vi "_Main_03.vi"() -> ()   [LabVIEW 2017]
uses:
  <vilib>/Instr/_visa.llb/VISA Configure Serial Port (Instr).vi
panel:
  out "Power LOG":cluster{dbl[], dbl[]}(graph)
  in  "Boolean":bool
  out "y":dbl
  in  "Set temp":dbl=195.0 min=195.0 max=395.0
  in  "OK Button":bool
  out "TrigTimer, s":dbl
  out "temp":dbl format="%#.2g"
  out "serv1":i32
  out "serv2":i32
  out "serv3":i32
  out "serv4":i32
  out "Vout, V":dbl format="%#.2g"
  out "Vin, V":dbl format="%#.3g"
  out "Temp, K":dbl
  out "Temp_sp, K":dbl
  out "Temp_gsp, K":dbl
  out "Temp LOG":cluster{dbl[], dbl[]}(graph)
  out "Bytes at Port":u32
  out "RecTry":i32
  in  "Stop Button":bool
  in  "COM port":refnum<visa-resource-name>
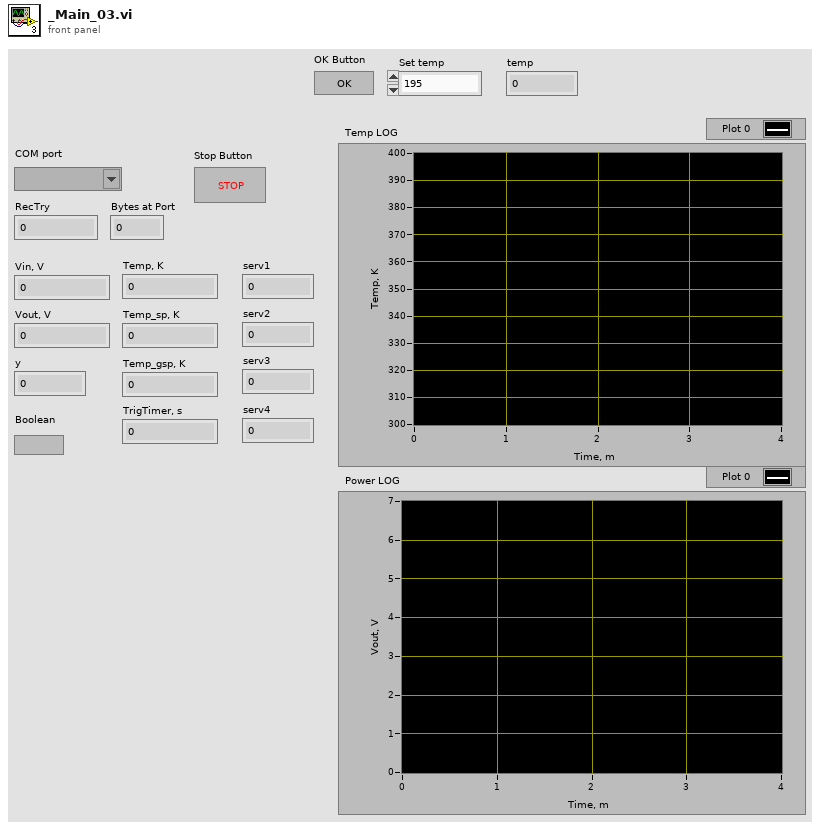
[diagram p1: front panel]
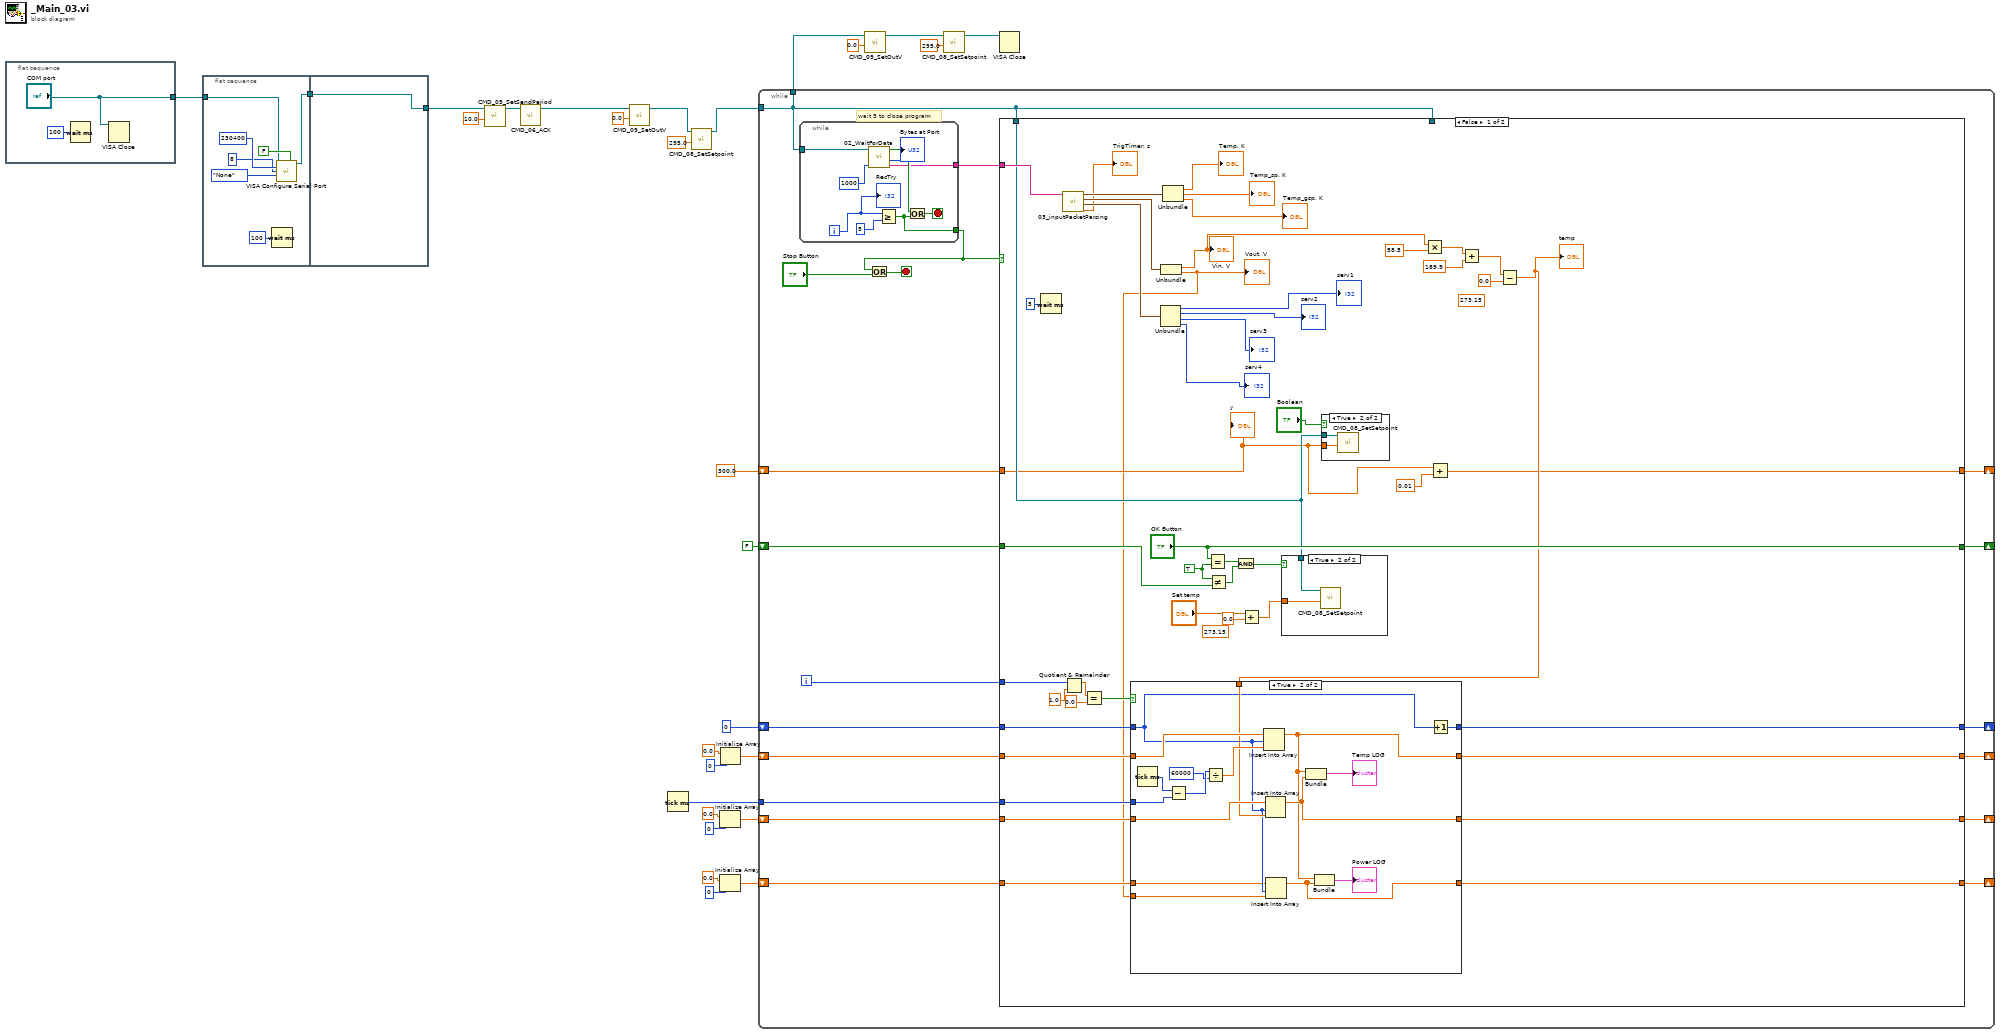
[diagram p0: block diagram]
diagram:
  n1 = flat-sequence {
    tunnel: ["COM port"] -> w28
    frame #0 {
      n2 = Wait (ms)(milliseconds to wait=u32 100) -> ()  [unwired: 1 out]
      n3 = VISA Close(VISA resource name="COM port") -> ()  [unwired: 1 in, 1 out]
    }
  }
  n4 = flat-sequence {
    tunnel: w28 -> [w33]
    tunnel: [w32] -> w25
    tunnel: [w38] -> w16
    tunnel: w25 -> [w38]
    frame #0 {
      n5 = Wait (ms)(milliseconds to wait=u32 100) -> ()  [unwired: 1 out]
      n6 = call-poly "VISA Configure Serial Port"("VISA resource name"=w33, "Enable Termination\nChar (T)"=FALSE ("Enable Termination\nChar (T)"), "baud rate (9600)"=u32 230400, "data bits (8)"=u16 8, "parity (0:none)"=enum16{"None", "Odd", "Even", "Mark", "Space"}."None") -> ("VISA resource name out"=w32:refnum<visa-resource-name>)  [unwired: 9 in, 1 out]
    }
    frame #1 {
    }
  }
  n7 = call "CMD_05_SetSendPeriod.vi"("Period, ms"=10.0, "VISA resource name"=w16) -> ("VISA resource name out"=w26:refnum<visa-resource-name>)  [unwired: 9 in]
  n8 = call "CMD_06_ACK.vi"("VISA resource name"=w26) -> ("VISA resource name out"=w12:refnum<visa-resource-name>)  [unwired: 10 in]
  n9 = call "CMD_09_SetOutV.vi"("Voltage, d"=0.0, "VISA resource name"=w12) -> ("VISA resource name out"=w11:refnum<visa-resource-name>)  [unwired: 9 in]
  n10 = Tick Count (ms)() -> (millisecond timer value=w20:u32)
  n11 = call "CMD_08_SetSetpoint.vi"("Setpoint, K"=295.0, "VISA resource name"=w11) -> ("VISA resource name out"=w10:refnum<visa-resource-name>)  [unwired: 9 in]
  n12 = Initialize Array(0.0 ("element"), 0 ("dimension size")) -> (w17:dbl[])
  n13 = Initialize Array(0.0 ("element"), 0 ("dimension size")) -> (w1:dbl[])
  n14 = Initialize Array(0.0 ("element"), 0 ("dimension size")) -> (w21:dbl[])
  n15 = while {
    tunnel: w10 -> [w43]
    tunnel: [w43] -> w15
    shift-right: [w52] -> _
    shift-left: 0 -> [w53]
    tunnel: w20 -> [w50]
    shift-right: [w48] -> _
    shift-left: w21 -> [w51]
    shift-right: [w47] -> _
    shift-left: w17 -> [w49]
    shift-right: [w45] -> _
    shift-left: FALSE ("OK Button") -> [w44]
    shift-right: [w41] -> _
    shift-left: 300.0 ("y") -> [w42]
    shift-right: [w39] -> _
    shift-left: w1 -> [w40]
    i -> [w54]
    stop <- w57 stop-if-true
    # "wait 5 to close program"
    n16 = while {
      tunnel: w43 -> [w138]
      tunnel: [w141] -> w56
      tunnel: [w142] -> w55
      i -> [w140]
      stop <- w144 stop-if-true
      n17 = call "02_WaitForData.vi"("WaitTimeoutMS"=u32 1000, "VISA"=w138) -> ("Buffer"=w142:string, "Bytes at Port"=→"Bytes at Port":u32, "Data Recived"=w143:bool)  [unwired: 7 in]
      n18 = Greater Or Equal?(x=w140, y=5) -> (x >= y?=w141:bool)
      n19 = Or(x=w143, y=w141) -> (x .or. y?=w144:bool)
      "RecTry" <- w140
    }
    n20 = Or(x=w56, y="Stop Button") -> (x .or. y?=w57:bool)
    n21 = case shown="False" w56 {
      tunnel: w55 -> [w97 _]
      tunnel: w54 -> [w103 _]
      tunnel: w43 -> [_ _]
      tunnel: w53 -> [w101 w137]
      tunnel: [w100 w137] -> w52
      tunnel: w51 -> [w80 w136]
      tunnel: w50 -> [w99 _]
      tunnel: w49 -> [w78 w135]
      tunnel: [w98 w136] -> w48
      tunnel: [w70 w135] -> w47
      tunnel: ["OK Button" w134] -> w45
      tunnel: w44 -> [w75 w134]
      tunnel: w43 -> [w65 _]
      tunnel: w42 -> [w63 w133]
      tunnel: [w64 w133] -> w41
      tunnel: w40 -> [w60 w132]
      tunnel: [w59 w132] -> w39
      frame False {
        (unwired) 273.15 ("y")
        w74 = TRUE ("x")
        (unwired) 273.15 ("y")
        n22 = Wait (ms)(milliseconds to wait=u32 5) -> ()  [unwired: 1 out]
        n23 = call "03_inputPacketParsing.vi"("string"=w97) -> ("TrigTimer, s"=→"TrigTimer, s":dbl, "Service"=w90:cluster{i32, i32, i32, i32}, "Voltage"=w91:cluster{dbl, dbl}, "Temp"=w95:cluster{dbl, dbl, dbl})  [unwired: 7 in]
        n24 = Quotient & Remainder(x=w103, y=1.0) -> (x-y*floor(x/y)=w106:dbl)  [unwired: 1 out]
        n25 = Equal?(x=w106, y=0.0) -> (x = y?=w102:bool)
        n26 = Unbundle(w90) -> (→"serv1":i32, →"serv2":i32, →"serv3":i32, →"serv4":i32)
        n27 = Unbundle(w91) -> (w85:dbl, w58:dbl)
        "Vin, V" <- w85
        "Vout, V" <- w58
        n28 = Unbundle(w95) -> (→"Temp, K":dbl, →"Temp_sp, K":dbl, →"Temp_gsp, K":dbl)
        n29 = Equal?(x="OK Button", y=w74) -> (x = y?=w77:bool)
        n30 = Not Equal?(x=w74, y=w75) -> (x != y?=w73:bool)
        n31 = And(x=w77, y=w73) -> (x .and. y?=w72:bool)
        n32 = Add(x="Set temp", y=0.0) -> (x+y=w69:dbl)
        n33 = case shown="True" w72 {
          tunnel: w69 -> [_ w110]
          tunnel: w65 -> [_ w109]
          frame False {
          }
          frame True {
            n34 = call "CMD_08_SetSetpoint.vi"("Setpoint, K"=w110, "VISA resource name"=w109) -> ()  [unwired: 9 in, 1 out]
          }
        }
        n35 = case shown="True" "Boolean" {
          tunnel: w65 -> [_ w108]
          tunnel: w63 -> [_ w107]
          frame False {
          }
          frame True {
            n36 = call "CMD_08_SetSetpoint.vi"("Setpoint, K"=w107, "VISA resource name"=w108) -> ()  [unwired: 9 in, 1 out]
          }
        }
        n37 = Multiply(x=w85, y=58.5) -> (x*y=w83:dbl)
        n38 = Add(x=w63, y=0.01) -> (x+y=w64:dbl)
        n39 = Add(x=w83, y=189.9) -> (x+y=w81:dbl)
        n40 = Subtract(x=w81, y=0.0) -> (x-y=w71:dbl)
        "temp" <- w71
        n41 = case shown="True" w102 {
          tunnel: w101 -> [w114 w120]
          tunnel: [w114 w127] -> w100
          tunnel: w80 -> [w112 w125]
          tunnel: w99 -> [_ w130]
          tunnel: w78 -> [w113 w124]
          tunnel: [w113 w122] -> w70
          tunnel: [w112 w118] -> w98
          tunnel: w71 -> [_ w121]
          tunnel: w60 -> [w111 w119]
          tunnel: [w111 w116] -> w59
          tunnel: w58 -> [_ w115]
          frame False {
          }
          frame True {
            n42 = Tick Count (ms)() -> (millisecond timer value=w131:u32)
            n43 = Subtract(x=w131, y=w130) -> (x-y=w129:u32)
            n44 = Divide(x=w129, y=u32 60000) -> (x/y=w126:dbl)
            n45 = Insert Into Array(array=w125, index=w120, new element=w126) -> (w118:dbl[])
            n46 = Insert Into Array(array=w124, index=w120, new element=w121) -> (w122:dbl[])
            n47 = Insert Into Array(array=w119, index=w120, new element=w115) -> (w116:dbl[])
            n48 = Bundle(w118, w122) -> (→"Temp LOG":cluster{dbl[], dbl[]})  [unwired: 1 in]
            n49 = Bundle(w118, w116) -> (→"Power LOG":cluster{dbl[], dbl[]})  [unwired: 1 in]
            n50 = Increment(x=w120) -> (x+1=w127:i32)
          }
        }
        "y" <- w63
      }
      frame True {
      }
    }
  }
  n51 = call "CMD_09_SetOutV.vi"("Voltage, d"=0.0, "VISA resource name"=w15) -> ("VISA resource name out"=w6:refnum<visa-resource-name>)  [unwired: 9 in]
  n52 = call "CMD_08_SetSetpoint.vi"("Setpoint, K"=295.0, "VISA resource name"=w6) -> ("VISA resource name out"=w5:refnum<visa-resource-name>)  [unwired: 9 in]
  n53 = VISA Close(VISA resource name=w5) -> ()  [unwired: 1 in, 1 out]
